vi "Get SMO RC Type.vi"(8 "error in (no error)":errorcluster, 11 "Instrument.sample-registry":refnum<class "Instrument.sample-registry.lvclass">) -> (0 "error out":errorcluster, 2 "Configuration.SMO.RC Type":T1=enum."STM", 3 "Instrument.sample-registry out":refnum<class "Instrument.sample-registry.lvclass">)   [LabVIEW 2019, in "Instrument.sample-registry.lvclass"]
uses:
  Instrument.sample-registry.lvclass
  <userlib>/LevyLab/Levylab Instruments/SMOs/RemoteControl/Typedefs/RC Com Type--enum.ctl
  <userlib>/LevyLab/Levylab Instruments/Instrument Types/VSource/Instrument.VSource.lvclass
  <userlib>/LevyLab/Levylab Instruments/SMOs/RemoteControl/RemoteControl.lvclass
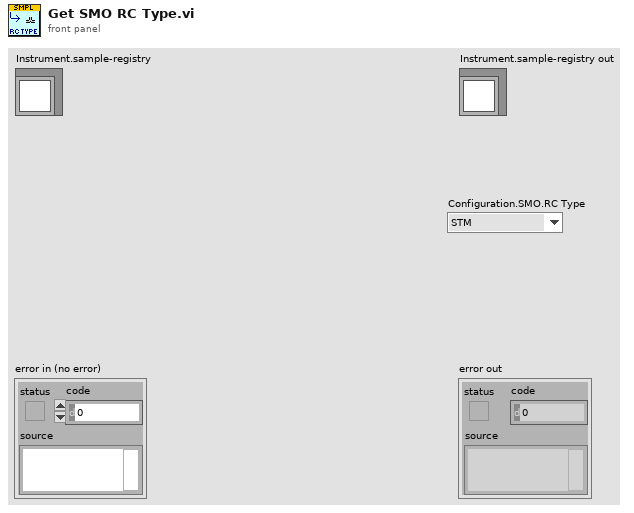
[diagram p1: front panel]
types:
  T1 = typedef "RemoteControl.lvclass/RC Com Type--enum.ctl" = enum16{"RC", "STM", "ZMQ"}
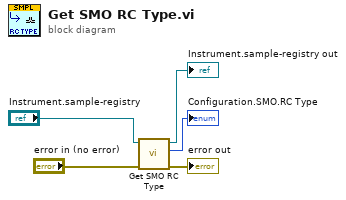
[diagram p0: block diagram]
diagram:
  n1 = call-parent "Get SMO RC Type.vi"("error in (no error)"="error in (no error)", "Instrument in"="Instrument.sample-registry") -> ("error out"=→"error out":errorcluster, "RC Type"=→"Configuration.SMO.RC Type":T1, "Instrument out"=→"Instrument.sample-registry out":refnum<class "Instrument.sample-registry.lvclass">)  [unwired: 7 in]
